vi "MRC Ds Comms Get Control Data With Joysticks.vi"(8 "error in (no error)":errorcluster) -> (0 "error out":errorcluster, 2 "joystickData out":T1, 3 "data out":T2)   [LabVIEW 2026, in "MrcLib.lvlib"]
doc: "MRC_Status MRC_CALLCONV MRC_DsComms_GetControlDataWithJoysticks(struct MRC_ControlData* data, struct MRC_Joysticks* joystickData);"
uses:
  MrcLib.lvlib
  MRC_ControlData.ctl
  MRC_Joysticks.ctl
  MrcLib.dll
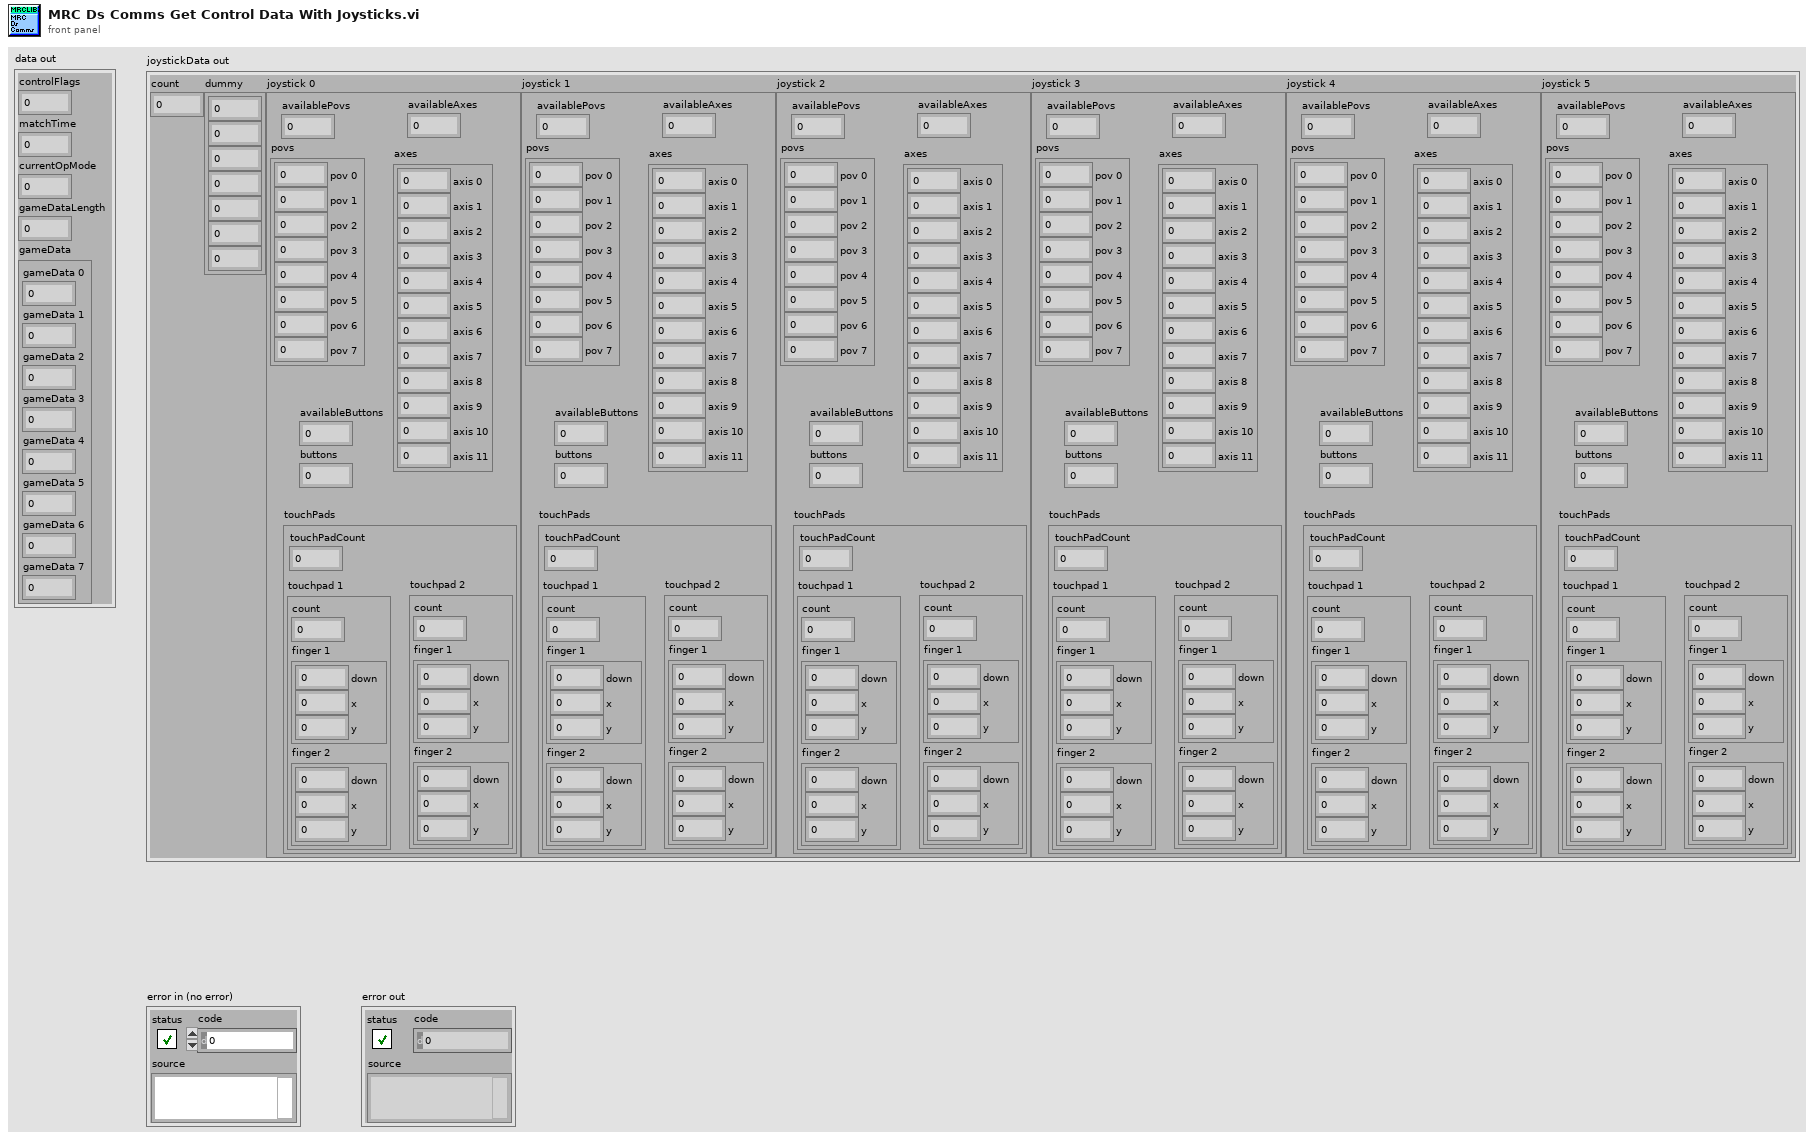
[diagram p1: front panel]
types:
  T1 = typedef "MrcLib.lvlib/MRC_Joysticks.ctl" = cluster{"count":u8, "dummy":cluster{i8, i8, i8, i8, i8, i8, i8}, "joystick 0":cluster{"availablePovs":u8, "povs":cluster{"pov 0":u8, "pov 1":u8, "pov 2":u8, "pov 3":u8, "pov 4":u8, "pov 5":u8, "pov 6":u8, "pov 7":u8}, "availableAxes":u16, "axes":cluster{"axis 0":i16, "axis 1":i16, "axis 2":i16, "axis 3":i16, "axis 4":i16, "axis 5":i16, "axis 6":i16, "axis 7":i16, "axis 8":i16, "axis 9":i16, "axis 10":i16, "axis 11":i16}, "availableButtons":u64, "buttons":u64, "touchPads":cluster{"touchPadCount":u8, "touchpad 1":cluster{"count":u8, "finger 1":cluster{"down":u8, "x":u16, "y":u16}, "finger 2":cluster{"down":u8, "x":u16, "y":u16}}, "touchpad 2":cluster{"count":u8, "finger 1":cluster{"down":u8, "x":u16, "y":u16}, "finger 2":cluster{"down":u8, "x":u16, "y":u16}}}}, "joystick 1":cluster{"availablePovs":u8, "povs":cluster{"pov 0":u8, "pov 1":u8, "pov 2":u8, "pov 3":u8, "pov 4":u8, "pov 5":u8, "pov 6":u8, "pov 7":u8}, "availableAxes":u16, "axes":cluster{"axis 0":i16, "axis 1":i16, "axis 2":i16, "axis 3":i16, "axis 4":i16, "axis 5":i16, "axis 6":i16, "axis 7":i16, "axis 8":i16, "axis 9":i16, "axis 10":i16, "axis 11":i16}, "availableButtons":u64, "buttons":u64, "touchPads":cluster{"touchPadCount":u8, "touchpad 1":cluster{"count":u8, "finger 1":cluster{"down":u8, "x":u16, "y":u16}, "finger 2":cluster{"down":u8, "x":u16, "y":u16}}, "touchpad 2":cluster{"count":u8, "finger 1":cluster{"down":u8, "x":u16, "y":u16}, "finger 2":cluster{"down":u8, "x":u16, "y":u16}}}}, "joystick 2":cluster{"availablePovs":u8, "povs":cluster{"pov 0":u8, "pov 1":u8, "pov 2":u8, "pov 3":u8, "pov 4":u8, "pov 5":u8, "pov 6":u8, "pov 7":u8}, "availableAxes":u16, "axes":cluster{"axis 0":i16, "axis 1":i16, "axis 2":i16, "axis 3":i16, "axis 4":i16, "axis 5":i16, "axis 6":i16, "axis 7":i16, "axis 8":i16, "axis 9":i16, "axis 10":i16, "axis 11":i16}, "availableButtons":u64, "buttons":u64, "touchPads":cluster{"touchPadCount":u8, "touchpad 1":cluster{"count":u8, "finger 1":cluster{"down":u8, "x":u16, "y":u16}, "finger 2":cluster{"down":u8, "x":u16, "y":u16}}, "touchpad 2":cluster{"count":u8, "finger 1":cluster{"down":u8, "x":u16, "y":u16}, "finger 2":cluster{"down":u8, "x":u16, "y":u16}}}}, "joystick 3":cluster{"availablePovs":u8, "povs":cluster{"pov 0":u8, "pov 1":u8, "pov 2":u8, "pov 3":u8, "pov 4":u8, "pov 5":u8, "pov 6":u8, "pov 7":u8}, "availableAxes":u16, "axes":cluster{"axis 0":i16, "axis 1":i16, "axis 2":i16, "axis 3":i16, "axis 4":i16, "axis 5":i16, "axis 6":i16, "axis 7":i16, "axis 8":i16, "axis 9":i16, "axis 10":i16, "axis 11":i16}, "availableButtons":u64, "buttons":u64, "touchPads":cluster{"touchPadCount":u8, "touchpad 1":cluster{"count":u8, "finger 1":cluster{"down":u8, "x":u16, "y":u16}, "finger 2":cluster{"down":u8, "x":u16, "y":u16}}, "touchpad 2":cluster{"count":u8, "finger 1":cluster{"down":u8, "x":u16, "y":u16}, "finger 2":cluster{"down":u8, "x":u16, "y":u16}}}}, "joystick 4":cluster{"availablePovs":u8, "povs":cluster{"pov 0":u8, "pov 1":u8, "pov 2":u8, "pov 3":u8, "pov 4":u8, "pov 5":u8, "pov 6":u8, "pov 7":u8}, "availableAxes":u16, "axes":cluster{"axis 0":i16, "axis 1":i16, "axis 2":i16, "axis 3":i16, "axis 4":i16, "axis 5":i16, "axis 6":i16, "axis 7":i16, "axis 8":i16, "axis 9":i16, "axis 10":i16, "axis 11":i16}, "availableButtons":u64, "buttons":u64, "touchPads":cluster{"touchPadCount":u8, "touchpad 1":cluster{"count":u8, "finger 1":cluster{"down":u8, "x":u16, "y":u16}, "finger 2":cluster{"down":u8, "x":u16, "y":u16}}, "touchpad 2":cluster{"count":u8, "finger 1":cluster{"down":u8, "x":u16, "y":u16}, "finger 2":cluster{"down":u8, "x":u16, "y":u16}}}}, "joystick 5":cluster{"availablePovs":u8, "povs":cluster{"pov 0":u8, "pov 1":u8, "pov 2":u8, "pov 3":u8, "pov 4":u8, "pov 5":u8, "pov 6":u8, "pov 7":u8}, "availableAxes":u16, "axes":cluster{"axis 0":i16, "axis 1":i16, "axis 2":i16, "axis 3":i16, "axis 4":i16, "axis 5":i16, "axis 6":i16, "axis 7":i16, "axis 8":i16, "axis 9":i16, "axis 10":i16, "axis 11":i16}, "availableButtons":u64, "buttons":u64, "touchPads":cluster{"touchPadCount":u8, "touchpad 1":cluster{"count":u8, "finger 1":cluster{"down":u8, "x":u16, "y":u16}, "finger 2":cluster{"down":u8, "x":u16, "y":u16}}, "touchpad 2":cluster{"count":u8, "finger 1":cluster{"down":u8, "x":u16, "y":u16}, "finger 2":cluster{"down":u8, "x":u16, "y":u16}}}}}
  T2 = typedef "MrcLib.lvlib/MRC_ControlData.ctl" = cluster{"controlFlags":u32, "matchTime":u16, "currentOpMode":u64, "gameDataLength":u8, "gameData":cluster{"gameData 0":u8, "gameData 1":u8, "gameData 2":u8, "gameData 3":u8, "gameData 4":u8, "gameData 5":u8, "gameData 6":u8, "gameData 7":u8}}
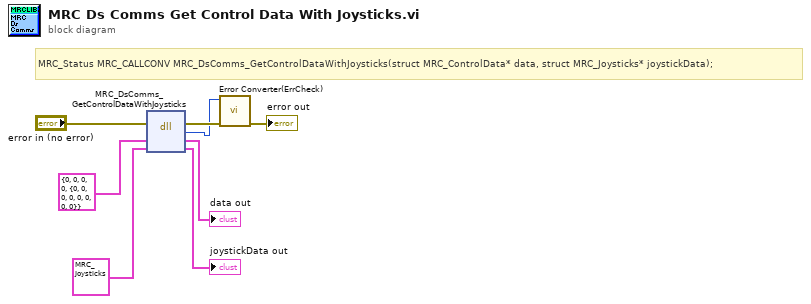
[diagram p0: block diagram]
diagram:
  # "MRC_Status MRC_CALLCONV MRC_DsComms_GetControlDataWithJoysticks(struct MRC_ControlData* data, struct MRC_Joysticks* joystickData);"
  n1 = dll-call lib="MrcLib.*" fn="MRC_DsComms_GetControlDataWithJoysticks"(error in="error in (no error)", "data"=T2 {"controlFlags"=0, "matchTime"=0, "currentOpMode"=0, "gameDataLength"=0, "gameData"={"gameData 0"=0, "gameData 1"=0, "gameData 2"=0, "gameData 3"=0, "gameData 4"=0, "gameData 5"=0, "gameData 6"=0, "gameData 7"=0}} ("data out"), "joystickData"=T1 {"count"=0, "dummy"={0, 0, 0, 0, 0, 0, 0}, "joystick 0"={"availablePovs"=0, "povs"={"pov 0"=0, "pov 1"=0, "pov 2"=0, "pov 3"=0, "pov 4"=0, "pov 5"=0, "pov 6"=0, "pov 7"=0}, "availableAxes"=0, "axes"={"axis 0"=0, "axis 1"=0, "axis 2"=0, "axis 3"=0, "axis 4"=0, "axis 5"=0, "axis 6"=0, "axis 7"=0, "axis 8"=0, "axis 9"=0, "axis 10"=0, "axis 11"=0}, "availableButtons"=0, "buttons"=0, "touchPads"={"touchPadCount"=0, "touchpad 1"={"count"=0, "finger 1"={"down"=0, "x"=0, "y"=0}, "finger 2"={"down"=0, "x"=0, "y"=0}}, "touchpad 2"={"count"=0, "finger 1"={"down"=0, "x"=0, "y"=0}, "finger 2"={"down"=0, "x"=0, "y"=0}}}}, "joystick 1"={"availablePovs"=0, "povs"={"pov 0"=0, "pov 1"=0, "pov 2"=0, "pov 3"=0, "pov 4"=0, "pov 5"=0, "pov 6"=0, "pov 7"=0}, "availableAxes"=0, "axes"={"axis 0"=0, "axis 1"=0, "axis 2"=0, "axis 3"=0, "axis 4"=0, "axis 5"=0, "axis 6"=0, "axis 7"=0, "axis 8"=0, "axis 9"=0, "axis 10"=0, "axis 11"=0}, "availableButtons"=0, "buttons"=0, "touchPads"={"touchPadCount"=0, "touchpad 1"={"count"=0, "finger 1"={"down"=0, "x"=0, "y"=0}, "finger 2"={"down"=0, "x"=0, "y"=0}}, "touchpad 2"={"count"=0, "finger 1"={"down"=0, "x"=0, "y"=0}, "finger 2"={"down"=0, "x"=0, "y"=0}}}}, "joystick 2"={"availablePovs"=0, "povs"={"pov 0"=0, "pov 1"=0, "pov 2"=0, "pov 3"=0, "pov 4"=0, "pov 5"=0, "pov 6"=0, "pov 7"=0}, "availableAxes"=0, "axes"={"axis 0"=0, "axis 1"=0, "axis 2"=0, "axis 3"=0, "axis 4"=0, "axis 5"=0, "axis 6"=0, "axis 7"=0, "axis 8"=0, "axis 9"=0, "axis 10"=0, "axis 11"=0}, "availableButtons"=0, "buttons"=0, "touchPads"={"touchPadCount"=0, "touchpad 1"={"count"=0, "finger 1"={"down"=0, "x"=0, "y"=0}, "finger 2"={"down"=0, "x"=0, "y"=0}}, "touchpad 2"={"count"=0, "finger 1"={"down"=0, "x"=0, "y"=0}, "finger 2"={"down"=0, "x"=0, "y"=0}}}}, "joystick 3"={"availablePovs"=0, "povs"={"pov 0"=0, "pov 1"=0, "pov 2"=0, "pov 3"=0, "pov 4"=0, "pov 5"=0, "pov 6"=0, "pov 7"=0}, "availableAxes"=0, "axes"={"axis 0"=0, "axis 1"=0, "axis 2"=0, "axis 3"=0, "axis 4"=0, "axis 5"=0, "axis 6"=0, "axis 7"=0, "axis 8"=0, "axis 9"=0, "axis 10"=0, "axis 11"=0}, "availableButtons"=0, "buttons"=0, "touchPads"={"touchPadCount"=0, "touchpad 1"={"count"=0, "finger 1"={"down"=0, "x"=0, "y"=0}, "finger 2"={"down"=0, "x"=0, "y"=0}}, "touchpad 2"={"count"=0, "finger 1"={"down"=0, "x"=0, "y"=0}, "finger 2"={"down"=0, "x"=0, "y"=0}}}}, "joystick 4"={"availablePovs"=0, "povs"={"pov 0"=0, "pov 1"=0, "pov 2"=0, "pov 3"=0, "pov 4"=0, "pov 5"=0, "pov 6"=0, "pov 7"=0}, "availableAxes"=0, "axes"={"axis 0"=0, "axis 1"=0, "axis 2"=0, "axis 3"=0, "axis 4"=0, "axis 5"=0, "axis 6"=0, "axis 7"=0, "axis 8"=0, "axis 9"=0, "axis 10"=0, "axis 11"=0}, "availableButtons"=0, "buttons"=0, "touchPads"={"touchPadCount"=0, "touchpad 1"={"count"=0, "finger 1"={"down"=0, "x"=0, "y"=0}, "finger 2"={"down"=0, "x"=0, "y"=0}}, "touchpad 2"={"count"=0, "finger 1"={"down"=0, "x"=0, "y"=0}, "finger 2"={"down"=0, "x"=0, "y"=0}}}}, "joystick 5"={"availablePovs"=0, "povs"={"pov 0"=0, "pov 1"=0, "pov 2"=0, "pov 3"=0, "pov 4"=0, "pov 5"=0, "pov 6"=0, "pov 7"=0}, "availableAxes"=0, "axes"={"axis 0"=0, "axis 1"=0, "axis 2"=0, "axis 3"=0, "axis 4"=0, "axis 5"=0, "axis 6"=0, "axis 7"=0, "axis 8"=0, "axis 9"=0, "axis 10"=0, "axis 11"=0}, "availableButtons"=0, "buttons"=0, "touchPads"={"touchPadCount"=0, "touchpad 1"={"count"=0, "finger 1"={"down"=0, "x"=0, "y"=0}, "finger 2"={"down"=0, "x"=0, "y"=0}}, "touchpad 2"={"count"=0, "finger 1"={"down"=0, "x"=0, "y"=0}, "finger 2"={"down"=0, "x"=0, "y"=0}}}}} ("joystickData in")) -> (error out=w3:errorcluster, "return type"=w1:i32, "data"=→"data out":T2, "joystickData"=→"joystickData out":T1)  [unwired: 2 in, 1 out]
  n2 = call "Error Converter(ErrCheck).vi"("error in (no error)"=w3, "status"=w1) -> ("error out"=→"error out":errorcluster)  [unwired: 9 in]
